vi "Draw Picture.vi"(10 "picture in":picture, 11 "Movable in":refnum<class "Movable.lvclass">) -> (2 "picture out":picture)   [LabVIEW 2024, in "Movable.lvclass"]
doc: "MIT Licence\nCopyright (c) 2024 David Grollier"
uses:
  Movable.lvclass
  Game Board Component.lvclass/Game Board Component.ctl
  Movable.lvclass/Movable.ctl
  Game Board Component.lvclass
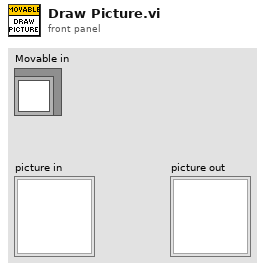
[diagram p1: front panel]
types:
  T1 = typedef "Coordinates.ctl" = cluster{"x":dbl, "y":dbl}
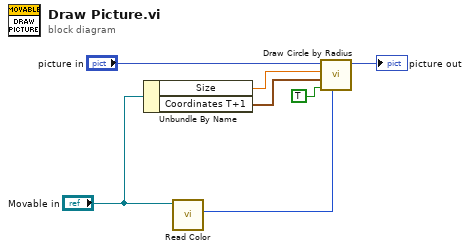
[diagram p0: block diagram]
diagram:
  n1 = Unbundle By Name("Movable in") -> ("Size"=w2:dbl, "Coordinates T+1"=w1:T1)
  n2 = call "Read Color.vi"("Game Board Component in"="Movable in") -> ("color"=w7:u32)  [unwired: 10 in]
  n3 = call <vilib>:"Draw Circle by Radius.vi"("color(black)"=w7, "fill?(F)"=TRUE, "pixel center"=w1, "radius"=w2, "picture"="picture in") -> ("new picture"=→"picture out":picture)  [unwired: 6 in]
